vi "Initialize AI Task.vi"(8 "error in (no error)":errorcluster, 11 "BNT_DMQmx-MCSV-TC in":refnum<class "BNT_DAQmx-MCSV-TC.lvclass">) -> (0 "error out":errorcluster, 3 "AI DAQmx Task":refnum<k21>)   [LabVIEW 2020, in "BNT_DAQmx.lvlib" / "BNT_DAQmx-MCSV-TC.lvclass"]
doc: "Initialize DAQmx Analog Input task.\n\n<b>Default Implementation:</b> Analog Input Voltage\n\nThis dynamic dispatch VI can be overritten by derived classes to implement other analog input tasks."
uses:
  BNT_DAQmx-MCSV-TC.lvclass
  C:/Users/holge/Documents/LVP/BNT/PGC/Packages/CSPP_Core/Actors/CSPP_BaseActor/CSPP_BaseActor.lvclass
  C:/Users/holge/Documents/LVP/BNT/PGC/Packages/BNT_DAQmx/BNT_DAQmx-MCSV/BNT_DAQmx-MCSV.lvclass
  CSPP_Core/Actors/CSPP_BaseActor/CSPP_BaseActor.lvclass/CSPP_BaseActor.ctl
  BNT_DAQmx-MCSV-TC.lvclass/BNT_DAQmx-MCSV-TC.ctl
  BNT_DAQmx-MCSV/BNT_DAQmx-MCSV.lvclass/BNT_DAQmx-MCSV.ctl
  CSPP_Core/Actors/CSPP_BaseActor/Read Object Name.vi
  Read CJC Channel.vi
  Read CJC Source.vi
  BNT_DAQmx-MCSV/Read AI Min.vi
  BNT_DAQmx-MCSV/Read AI Max.vi
  BNT_DAQmx-MCSV/Read AI DAQmx Physical Channels.vi
  Read Thermocouple Type.vi
  Read CJC Value.vi
  <vilib>/DAQmx/create/channels.llb/DAQmx Create Channel (AI-Temperature-Thermocouple).vi
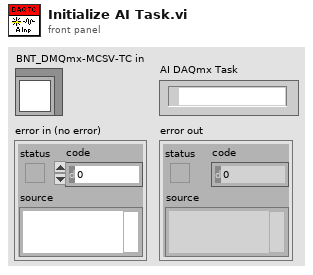
[diagram p1: front panel]
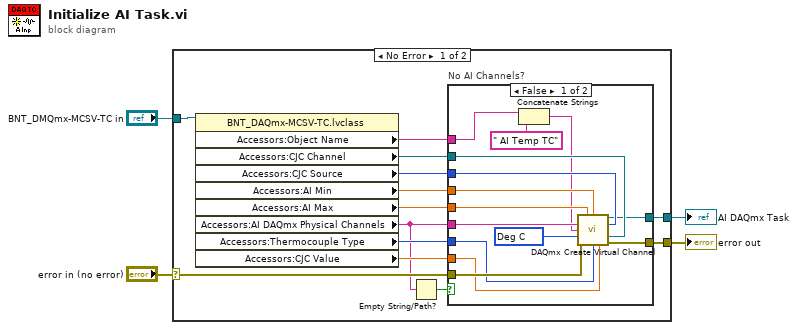
[diagram p0: block diagram]
diagram:
  n1 = case shown="No Error" "error in (no error)" {
    selector: "error in (no error)" -> [w17 w33]
    tunnel: [w8 w33] -> w3
    tunnel: "BNT_DMQmx-MCSV-TC in" -> [w16 _]
    tunnel: [w9 _] -> w1
    frame No Error {
      n2 = property class="BNT_DAQmx-MCSV-TC.lvclass"(reference=w16) -> ("Accessors:Object Name"=w7:string, "Accessors:CJC Channel"=w12:refnum<k21>, "Accessors:CJC Source"=w13:i32, "Accessors:AI Min"=w14:dbl, "Accessors:AI Max"=w15:dbl, "Accessors:AI DAQmx Physical Channels"=w6:tag, "Accessors:Thermocouple Type"=w11:i32, "Accessors:CJC Value"=w10:dbl)  [unwired: 1 in, 2 out]
      n3 = Empty String/Path?(string/path=w6) -> (empty?=w5:bool)
      n4 = case "No AI Channels?" shown="False" w5 {
        tunnel: w17 -> [w31 w32]
        tunnel: w6 -> [w30 _]
        tunnel: w15 -> [w29 _]
        tunnel: w14 -> [w28 _]
        tunnel: w13 -> [w26 _]
        tunnel: w12 -> [w25 _]
        tunnel: w11 -> [w24 _]
        tunnel: w10 -> [w23 _]
        tunnel: [w22 _] -> w9
        tunnel: [w21 w32] -> w8
        tunnel: w7 -> [w19 _]
        frame False {
          w27 = 10143 items=["Deg C"=10143, "Deg F"=10144, "Kelvins"=10325, "Deg R"=10145, "From Custom Scale"=10065] ("units")
          n5 = Concatenate Strings(w19, " AI Temp TC" ("string")) -> (w18:string)
          n6 = call-poly <vilib>:"DAQmx Create Virtual Channel.vi"("maximum value"=w29, "minimum value"=w28, "physical channels"=w30, "cjc source"=w26, "name to assign"=w18, "units"=w27, "cjc channel"=w25, "error in"=w31, "thermocouple type"=w24, "cjc value"=w23) -> ("task out"=w22:refnum<k21>, "error out"=w21:errorcluster)  [unwired: 4 in]
        }
        frame True {
        }
      }
    }
    frame Error {
    }
  }
  "error out" <- w3
  "AI DAQmx Task" <- w1
